vi "Update DER_Status in Listbox.vi"(4 "Mode Column":i32, 6 "VF Column":i32, 7 "DevIDs in Config":T1[](array[typedef]), 9 "DER_Status (Array)":T2[](array[typedef]), 11 "MulticolumnListbox in":refnum<vi>) -> ()   [LabVIEW 2018, in "EMS User Interface Actor.lvlib" / "EMS User Interface.lvclass"]
uses:
  EMS User Interface.lvclass
  <vilib>/ORNL/CSEISMIC DDS/CSEISMIC DDS Base/Data Types/DER_Status.ctl
  <vilib>/ORNL/CSEISMIC DDS/CSEISMIC DDS Base/Data Types/Controls/DeviceID.ctl
  <vilib>/ORNL/CSEISMIC DDS/CSEISMIC DDS Base/Data Types/Controls/DroopCurve.ctl
  <vilib>/Utility/miscctls.llb/LVRowAndColumnTypeDef.ctl
  <vilib>/ORNL/CSEISMIC DDS/CSEISMIC DDS Base/CSEISMIC DDS.lvclass
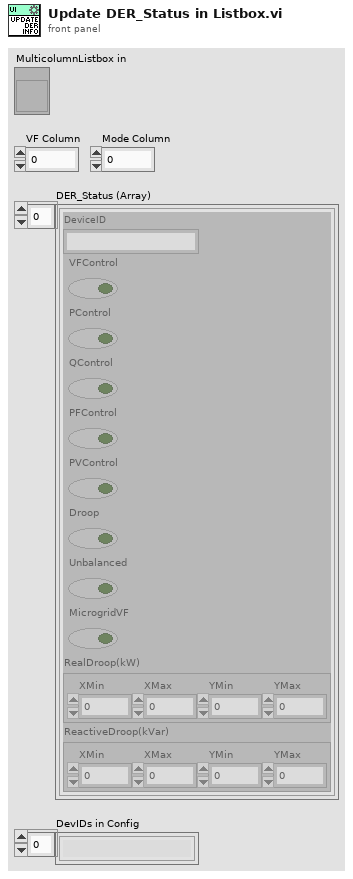
[diagram p1: front panel]
types:
  T1 = typedef "CSEISMIC DDS.lvlib/CSEISMIC DDS.lvclass/DeviceID.ctl" = string
  T2 = typedef "CSEISMIC DDS.lvlib/CSEISMIC DDS.lvclass/DER_Status.ctl" = cluster{"DeviceID":T1, "VFControl":bool, "PControl":bool, "QControl":bool, "PFControl":bool, "PVControl":bool, "Droop":bool, "Unbalanced":bool, "MicrogridVF":bool, "RealDroop(kW)":T3, "ReactiveDroop(kVar)":T3}
  T3 = typedef "CSEISMIC DDS.lvlib/CSEISMIC DDS.lvclass/DroopCurve.ctl" = cluster{"XMin":dbl, "XMax":dbl, "YMin":dbl, "YMax":dbl}
  T4 = typedef "LVRowAndColumnTypeDef.ctl" = cluster{"Row":i32, "Column":i32}
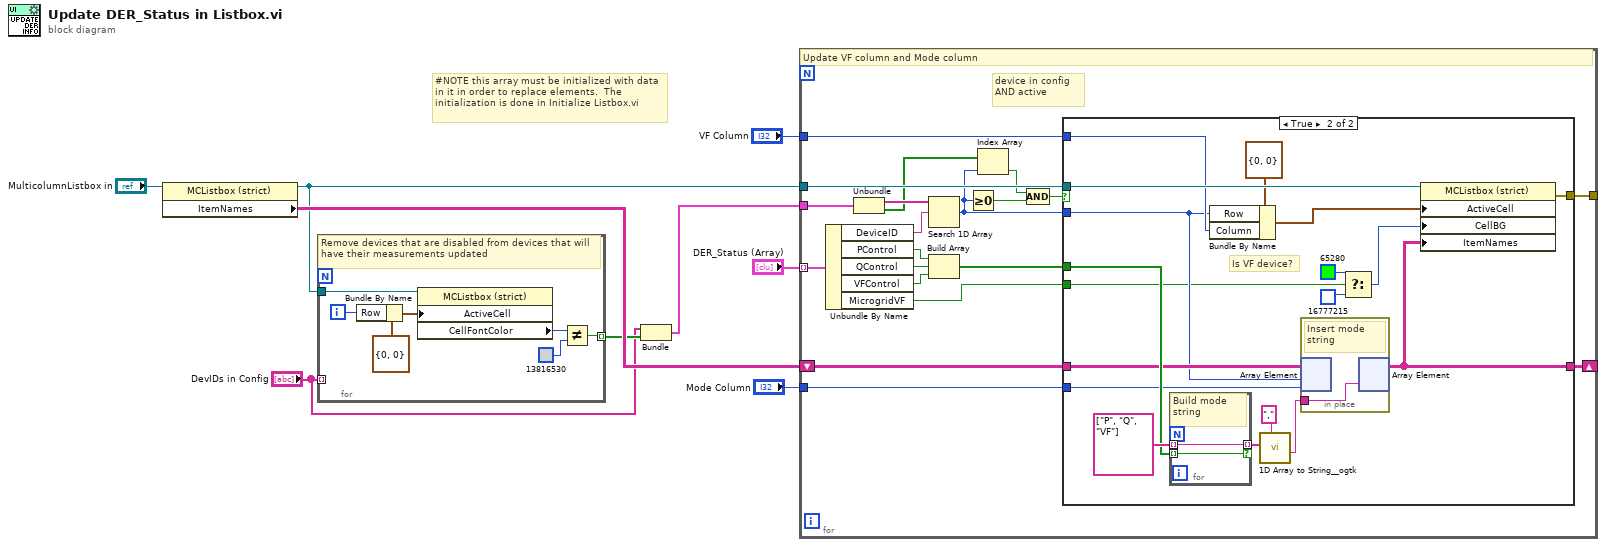
[diagram p0: block diagram]
diagram:
  # "#NOTE this array must be initialized with data in it in order to replace elements.  The initialization is done in Initialize Listbox.vi"
  n1 = property class="MCListbox (strict)"(reference="MulticolumnListbox in") -> (reference out=w4:refnum<vi>, "ItemNames"=w5:string[][])  [unwired: 1 in, 1 out]
  n2 = for {
    tunnel: "DevIDs in Config" -> [_] mode=indexing
    tunnel: w4 -> [w16]
    tunnel: [w10] -> w3 mode=indexing
    i -> [w13]
    # "Remove devices that are disabled from devices that will have their measurements updated"
    n3 = Bundle By Name(cluster=T4 {"Row"=0, "Column"=0} ("Active Cell:Active Cell"), "Row"=w13) -> (w14:T4)
    n4 = property on="Property Node" class="MCListbox (strict)"(reference=w16, "ActiveCell"=w14) -> ("CellFontColor"=w12:u32)  [unwired: 1 in, 2 out]
    n5 = Not Equal?(x=w12, y=u32 13816530) -> (x != y?=w10:bool)
  }
  n6 = Bundle("DevIDs in Config"="DevIDs in Config", w3) -> (w1:cluster{"DevIDs in Config":T1[], bool[]})  [unwired: 1 in]
  n7 = for {
    tunnel: w1 -> [w29]
    tunnel: "DER_Status (Array)" -> [w35] mode=indexing
    tunnel: w4 -> [w36]
    tunnel: "VF Column" -> [w28]
    tunnel: "Mode Column" -> [w26]
    shift-right: [w25] -> _
    shift-left: w5 -> [w27]
    tunnel: [w23] -> _
    # "device in config AND active"
    # "Update VF column and Mode column"
    n8 = Unbundle By Name(w35) -> ("DeviceID"=w34:T1, "PControl"=w33:bool, "QControl"=w32:bool, "VFControl"=w31:bool, "MicrogridVF"=w24:bool)
    n9 = Unbundle(w29) -> ("DevIDs in Config"=w22:T1[], w19:bool[])
    n10 = Search 1D Array(1D array=w22, element=w34) -> (index of element=w18:i32)  [unwired: 1 in]
    n11 = Build Array(w33, w32, w31) -> (w30:bool[])
    n12 = Greater Or Equal To 0?(x=w18) -> (x >= 0?=w21:bool)
    n13 = Index Array(array=w19, index=w18) -> (element=w20:bool)
    n14 = Compound Arithmetic op=AND(w20, w21) -> (w17:bool)
    n15 = case shown="True" w17 {
      tunnel: w36 -> [_ w55]
      tunnel: w30 -> [_ w46]
      tunnel: w28 -> [_ w45]
      tunnel: w27 -> [w37 w44]
      tunnel: w18 -> [_ w43]
      tunnel: w26 -> [_ w42]
      tunnel: [w37 w40] -> w25
      tunnel: w24 -> [_ w39]
      tunnel: [_ w38] -> w23
      frame False {
      }
      frame True {
        # "Is VF device?"
        n16 = for {
          tunnel: string[] ["P", "Q", "VF"] -> [w58] mode=indexing
          tunnel: w46 -> [w57] mode=indexing
          tunnel: [w58] -> w48 mode=indexing if=w57
          # "Build mode string"
        }
        n17 = Bundle By Name(cluster=T4 {"Row"=0, "Column"=0} ("Active Cell:Active Cell"), "Row"=w43, "Column"=w45) -> (w53:T4)
        n18 = call <userlib>:"1D Array to String__ogtk.vi"("delimiter (Tab)"=",", "Array of Strings"=w48) -> ("delimited string"=w41:string)  [unwired: 9 in]
        n19 = in-place {
          in-place-border: w41 -> [w56]
          # "Insert mode string"
          n20 = in-place-array #1(w44, w43, w42) -> ()  [unwired: 1 out]
          n21 = in-place-array #1(w56) -> (w40:string[][])  [unwired: 2 out]
        }
        n22 = Select(t=u32 65280, s=w39, f=u32 16777215) -> (s? t:f=w50:u32)
        n23 = property on="Property Node" class="MCListbox (strict)"(reference=w55, "ActiveCell"=w53, "CellBG"=w50, "ItemNames"=w40) -> (error out=w38:errorcluster)  [unwired: 1 in, 1 out]
      }
    }
  }
